vi "ConfigParseProgram.vi"(8 "error in (no error)":errorcluster, 10 "node result array":refnum<k20>[](array[refnum])) -> (0 "error out":errorcluster, 3 "Program Array":string[][](array[string]))   [LabVIEW 2018, in "Config.lvlib"]
uses:
  Config.lvlib
  <vilib>/xml/NI_XML.lvlib
  <resource>/objmgr/DOMUserDefRef.rc
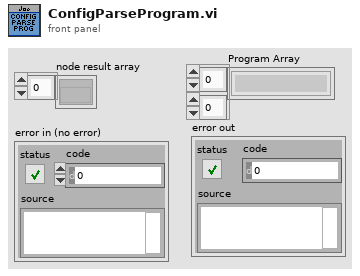
[diagram p1: front panel]
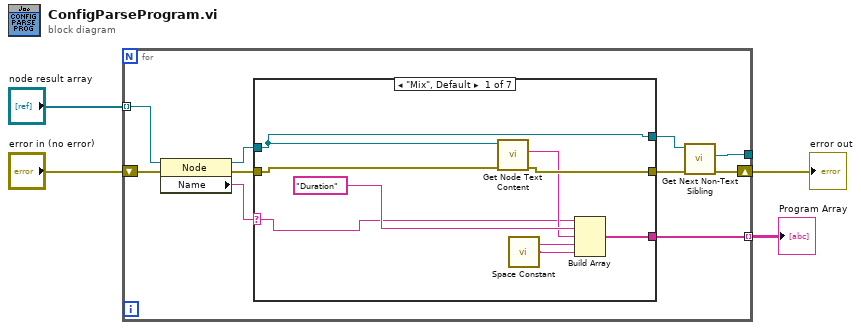
[diagram p0: block diagram]
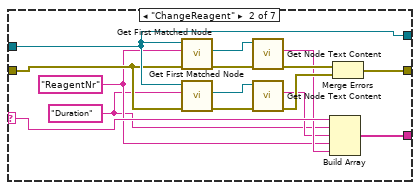
[diagram p2: hidden frame]
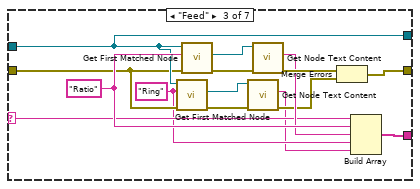
[diagram p3: hidden frame]
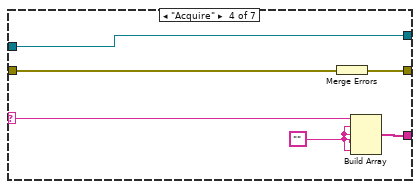
[diagram p4: hidden frame]
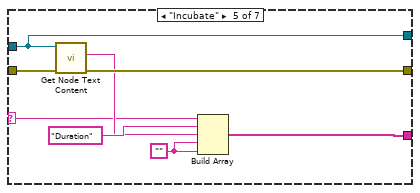
[diagram p5: hidden frame]
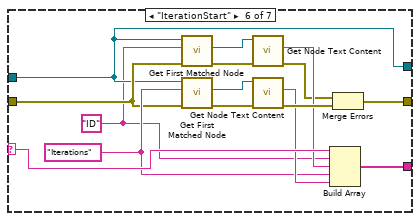
[diagram p6: hidden frame]
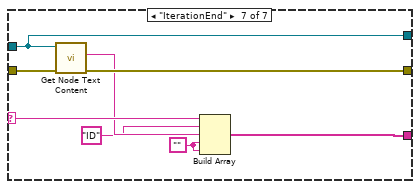
[diagram p7: hidden frame]
diagram:
  n1 = for {
    shift-right: [w5] -> w1
    shift-left: "error in (no error)" -> [w10]
    tunnel: [w6] -> w2 mode=indexing
    tunnel: "node result array" -> [w14] mode=indexing
    tunnel: [w7] -> _
    n2 = property class="Node"(reference=w14, error in=w10) -> (reference out=w11:refnum<k20>, error out=w12:errorcluster, "Name"=w13:string)
    n3 = case shown="\"Mix\", Default" w13 {
      selector: w13 -> [w17 w28 w46 w56 w63 w77 w87]
      tunnel: w12 -> [w21 w36 w41 w54 w60 w71 w85]
      tunnel: w11 -> [w22 w37 w42 w58 w61 w70 w86]
      tunnel: [w22 w37 w42 w58 w61 w70 w86] -> w9
      tunnel: [w20 w29 w49 w57 w66 w78 w84] -> w8
      tunnel: [w16 w27 w45 w55 w62 w76 w89] -> w6
      frame "Mix", Default {
        n4 = call <vilib>:"Get Node Text Content.vi"("error in (no error)"=w21, "node in"=w22) -> ("error out"=w20:errorcluster, "node text"=w18:string)  [unwired: 7 in, 1 out]
        n5 = call <vilib>:"Space Constant.vi"() -> ("String"=w15:string)
        n6 = Build Array(w17, "Duration" ("XPath expression"), w18, w15, w15) -> (w16:string[])
      }
      frame "ChangeReagent" {
        w23 = "Duration" ("XPath expression")
        w25 = "ReagentNr" ("XPath expression")
        n7 = call <vilib>:"Get First Matched Node.vi"("error in (no error)"=w36, "XPath expression"=w25, "node in"=w37) -> ("error out"=w35:errorcluster, "node result"=w34:refnum<k20>)  [unwired: 6 in, 1 out]
        n8 = call <vilib>:"Get First Matched Node.vi"("error in (no error)"=w36, "XPath expression"=w23, "node in"=w37) -> ("error out"=w33:errorcluster, "node result"=w32:refnum<k20>)  [unwired: 6 in, 1 out]
        n9 = call <vilib>:"Get Node Text Content.vi"("error in (no error)"=w35, "node in"=w34) -> ("error out"=w31:errorcluster, "node text"=w26:string)  [unwired: 7 in, 1 out]
        n10 = call <vilib>:"Get Node Text Content.vi"("error in (no error)"=w33, "node in"=w32) -> ("error out"=w30:errorcluster, "node text"=w24:string)  [unwired: 7 in, 1 out]
        n11 = Build Array(w28, w23, w24, w25, w26) -> (w27:string[])
        n12 = Merge Errors(w31, w30) -> (w29:errorcluster)
      }
      frame "Feed" {
        w39 = "Ring" ("XPath expression")
        w48 = "Ratio" ("XPath expression")
        n13 = call <vilib>:"Get First Matched Node.vi"("error in (no error)"=w41, "XPath expression"=w39, "node in"=w42) -> ("error out"=w44:errorcluster, "node result"=w43:refnum<k20>)  [unwired: 6 in, 1 out]
        n14 = call <vilib>:"Get First Matched Node.vi"("error in (no error)"=w41, "XPath expression"=w48, "node in"=w42) -> ("error out"=w52:errorcluster, "node result"=w51:refnum<k20>)  [unwired: 6 in, 1 out]
        n15 = call <vilib>:"Get Node Text Content.vi"("error in (no error)"=w44, "node in"=w43) -> ("error out"=w40:errorcluster, "node text"=w38:string)  [unwired: 7 in, 1 out]
        n16 = call <vilib>:"Get Node Text Content.vi"("error in (no error)"=w52, "node in"=w51) -> ("error out"=w50:errorcluster, "node text"=w47:string)  [unwired: 7 in, 1 out]
        n17 = Merge Errors(w50, w40) -> (w49:errorcluster)
        n18 = Build Array(w46, w48, w47, w39, w38) -> (w45:string[])
      }
      frame "Acquire" {
        w53 = ""
        n19 = Merge Errors(w54) -> (w57:errorcluster)
        n20 = Build Array(w56, w53, w53, w53, w53) -> (w55:string[])
      }
      frame "Incubate" {
        w59 = "" ("element")
        n21 = call <vilib>:"Get Node Text Content.vi"("error in (no error)"=w60, "node in"=w61) -> ("error out"=w66:errorcluster, "node text"=w64:string)  [unwired: 7 in, 1 out]
        n22 = Build Array(w63, "Duration" ("XPath expression"), w64, w59, w59) -> (w62:string[])
      }
      frame "IterationStart" {
        w68 = "ID" ("XPath expression")
        w74 = "Iterations" ("XPath expression")
        n23 = call <vilib>:"Get First Matched Node.vi"("error in (no error)"=w71, "XPath expression"=w68, "node in"=w70) -> ("error out"=w73:errorcluster, "node result"=w72:refnum<k20>)  [unwired: 6 in, 1 out]
        n24 = call <vilib>:"Get First Matched Node.vi"("error in (no error)"=w71, "XPath expression"=w74, "node in"=w70) -> ("error out"=w81:errorcluster, "node result"=w80:refnum<k20>)  [unwired: 6 in, 1 out]
        n25 = call <vilib>:"Get Node Text Content.vi"("error in (no error)"=w73, "node in"=w72) -> ("error out"=w67:errorcluster, "node text"=w69:string)  [unwired: 7 in, 1 out]
        n26 = call <vilib>:"Get Node Text Content.vi"("error in (no error)"=w81, "node in"=w80) -> ("error out"=w79:errorcluster, "node text"=w75:string)  [unwired: 7 in, 1 out]
        n27 = Build Array(w77, w68, w69, w74, w75) -> (w76:string[])
        n28 = Merge Errors(w67, w79) -> (w78:errorcluster)
      }
      frame "IterationEnd" {
        w88 = ""
        n29 = call <vilib>:"Get Node Text Content.vi"("error in (no error)"=w85, "node in"=w86) -> ("error out"=w84:errorcluster, "node text"=w83:string)  [unwired: 7 in, 1 out]
        n30 = Build Array(w87, "ID", w83, w88, w88) -> (w89:string[])
      }
    }
    n31 = call <vilib>:"Get Next Non-Text Sibling.vi"("error in (no error)"=w8, "node in"=w9) -> ("error out"=w5:errorcluster, "sibling node"=w7:refnum<k20>)  [unwired: 6 in, 2 out]
  }
  "Program Array" <- w2
  "error out" <- w1
